vi "Handle Exception.vi"(7 "Processing In":refnum<class "Processing.lvclass">, 8 "error in (no error)":errorcluster, 11 "TestCSRFController in":refnum<class "TestCSRFController.lvclass">) -> (0 "error out":errorcluster, 5 "Processing":refnum<class "Processing.lvclass">)   [LabVIEW 2020, in "TestCSRFController.lvclass"]
uses:
  TestCSRFController.lvclass
  <vilib>/IlluminatedG/IG HTTP Server/HTTP Server/Processing/Processing.lvclass
  <vilib>/IlluminatedG/IG HTTP Server/HTTP Server/Processing/Processing.lvclass/Processing.ctl
  <vilib>/IlluminatedG/IG HTTP Utils/HTTP Utils/Redirect Response/Redirect Response.lvclass
  C:/Program Files (x86)/National Instruments/LabVIEW 2020/vi.lib/IlluminatedG/IG HTTP Utils/HTTP Utils/Response/Response.lvclass
  <vilib>/IlluminatedG/lv-stream/URI/URI.lvclass
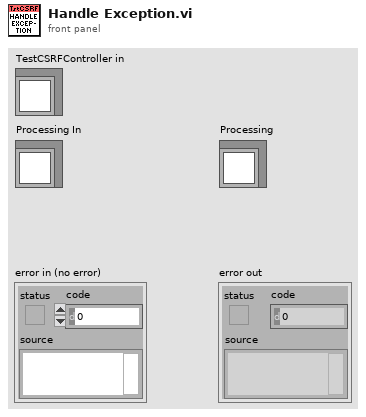
[diagram p1: front panel]
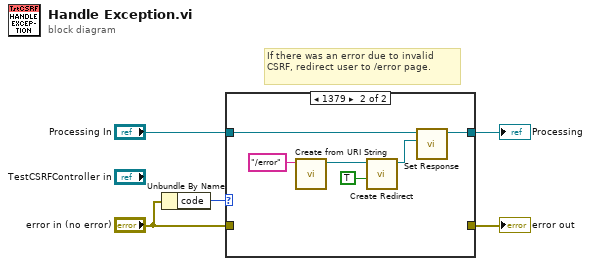
[diagram p0: block diagram]
diagram:
  # "If there was an error due to invalid CSRF, redirect user to /error page."
  n1 = Unbundle By Name("error in (no error)") -> ("code"=w5:i32)
  n2 = case shown="1379" w5 {
    tunnel: "Processing In" -> [w6 w12]
    tunnel: "error in (no error)" -> [w7 _]
    tunnel: [w7 _] -> w2
    tunnel: [w6 w11] -> w1
    frame Default {
    }
    frame 1379 {
      n3 = call <vilib>:"Create from URI String.vi"("URI String"="/error") -> ("URI out"=w10:refnum<class "URI.lvclass">)  [unwired: 9 in, 1 out]
      n4 = call <vilib>:"Create Redirect.vi"("Force GET? (F)"=TRUE, "Redirect URI"=w10) -> ("Redirect Response out"=w8:refnum<class "Redirect Response.lvclass">)  [unwired: 8 in, 1 out]
      n5 = call <vilib>:"Set Response.vi"("Response"=w8, "Processing in"=w12) -> ("Processing out"=w11:refnum<class "Processing.lvclass">)  [unwired: 9 in]
    }
  }
  "error out" <- w2
  "Processing" <- w1
